vi "UArrNum Pathogorean Theorem.vi"(9 "Coordinates":i32[](array[numeric])) -> (3 "Segment Length":dbl format="%.2f")   [LabVIEW 2013]
doc: "Given a coordinate array in standard IMAQ format, (X1,Y1,X2,Y2) this vi will calculate the length of the segment defined by the endpoints."
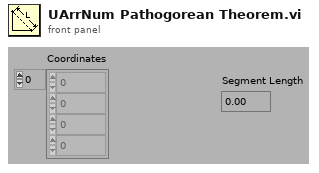
[diagram p1: front panel]
types:
  T1 = cluster{"[0]":dbl, "[1]":dbl, "[2]":dbl, "[3]":dbl}
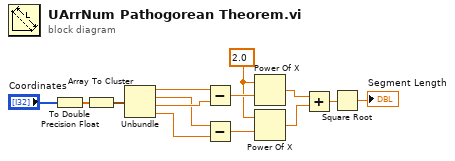
[diagram p0: block diagram]
diagram:
  w7 = 2.0 ("y")
  n1 = To Double Precision Float(number="Coordinates") -> (double precision float=w8:dbl[])
  n2 = Array To Cluster(array=w8) -> (cluster=w13:T1)
  n3 = Unbundle(w13) -> ("[0]"=w12:dbl, "[1]"=w5:dbl, "[2]"=w11:dbl, "[3]"=w10:dbl)
  n4 = Subtract(x=w12, y=w11) -> (x-y=w9:dbl)
  n5 = Subtract(x=w5, y=w10) -> (x-y=w6:dbl)
  n6 = Power Of X(1:w9, 2:w7) -> (0:w4:dbl)
  n7 = Power Of X(1:w6, 2:w7) -> (0:w3:dbl)
  n8 = Add(x=w4, y=w3) -> (x+y=w2:dbl)
  n9 = Square Root(x=w2) -> (sqrt(x)=→"Segment Length":dbl)
